vi "fgv_FOV.vi"(8 "error in":errorcluster, 11 "Function":T2) -> (0 "error out":errorcluster, 1 "Objectives (section names)":string[](array[string]), 2 "Data (Format B)":cluster{"FOV setup":T1}[](array[cluster]), 3 "Data (Format A)":T3(array[cluster]))   [LabVIEW 2020]
uses:
  Typedefs/FOV FGV states.ctl
  <vilib>/Utility/miscctls.llb/LVStringsAndValuesArrayTypeDef_SGL.ctl
  Typedefs/Which path.ctl
  <vilib>/Utility/config.llb/Read Key (Double).vi
  <vilib>/Utility/config.llb/NI_LVConfig.lvlib
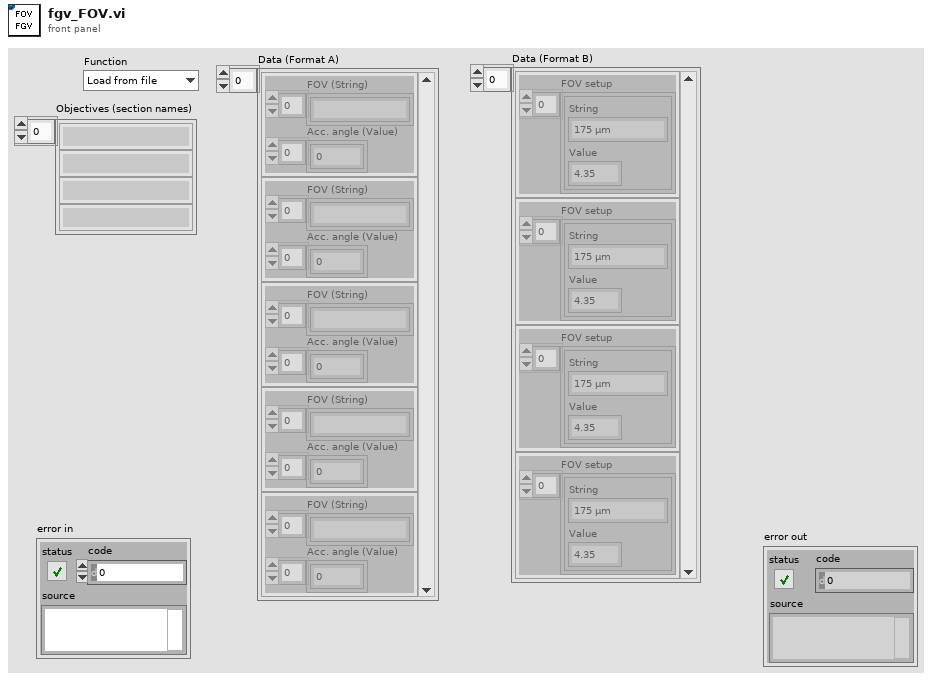
[diagram p1: front panel]
types:
  T1 = typedef "LVStringsAndValuesArrayTypeDef_SGL.ctl" = cluster{"String":string, "Value":sgl}[]
  T2 = typedef "FOV FGV states.ctl" = enum16{"Load from file", "Read FGV", "Update section name", "Delete section", "Add section", "Cleanup ini file"}
  T3 = cluster{"FOV (String)":string[], "Acc. angle (Value)":dbl[]}[]
  T4 = typedef "Which path.ctl" = enum16{"Configuration Files", "Calibration Files", "Images", "Setup.ini", "Loaded User profile.ini", "User's-Previous session.ini", "New user profile.ini", "Selected User profile.ini", "User profiles folder", "Power meter scaling.txt", "FOV Cal.ini", "Calibration.ini"}
  T5 = typedef "NI_LVConfig.lvlib/Config Data RefNum.ctl" = refnum<k1>
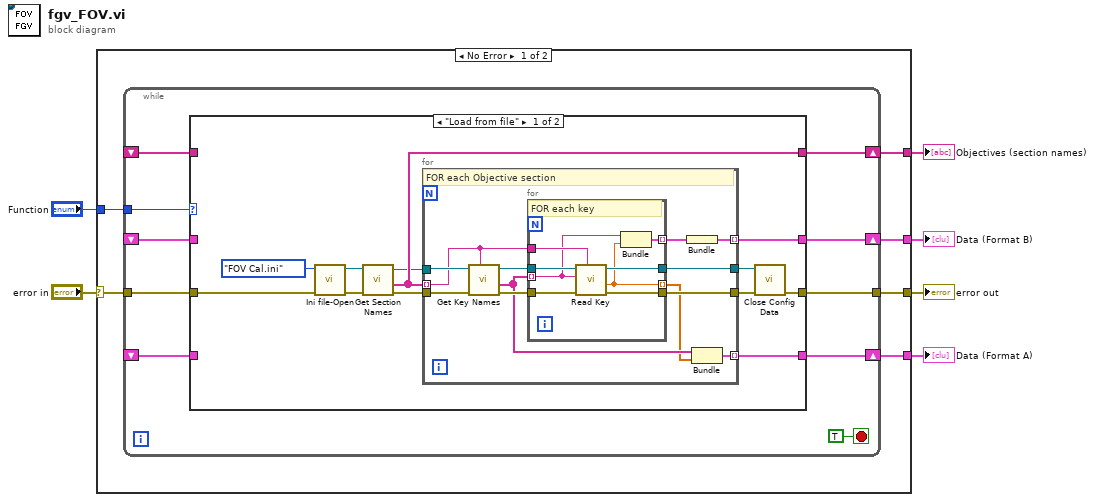
[diagram p0: block diagram]
diagram:
  n1 = case shown="No Error" "error in" {
    selector: "error in" -> [w8 w59]
    tunnel: "Function" -> [w12 _]
    tunnel: [w11 _] -> w5
    tunnel: [w10 _] -> w4
    tunnel: [w9 w59] -> w2
    tunnel: [w7 _] -> w1
    frame No Error {
      n2 = while {
        shift-right: [w22] -> w10
        shift-left: _ -> [w18]
        shift-right: [w21] -> w11
        shift-left: _ -> [w17]
        tunnel: w12 -> [w19]
        tunnel: [w16] -> w9
        tunnel: w8 -> [w15]
        shift-right: [w14] -> w7
        shift-left: _ -> [w13]
        stop <- TRUE stop-if-true
        n3 = case shown="\"Load from file\"" w19 {
          tunnel: [w34 w58] -> w22
          tunnel: [w31 w57] -> w21
          tunnel: w18 -> [_ w58]
          tunnel: w17 -> [_ w57]
          tunnel: [w25 w56] -> w16
          tunnel: w15 -> [w24 w56]
          tunnel: [w23 w55] -> w14
          tunnel: w13 -> [_ w55]
          frame "Load from file" {
            n4 = call "Ini file-Open.vi"("Error In"=w24, "Which file?"=Which_path."FOV Cal.ini") -> ("error out"=w29:errorcluster, "User profile ini file ref"=w28:T5)  [unwired: 6 in, 2 out]
            n5 = call <vilib>:"Get Section Names.vi"("error in (no error)"=w29, "refnum"=w28) -> ("error out"=w32:errorcluster, "section names"=w34:string[], "refnum out"=w33:T5)  [unwired: 7 in]
            n6 = for {
              tunnel: w34 -> [w42] mode=indexing
              tunnel: w33 -> [w46]
              tunnel: [w43] -> w27
              tunnel: w32 -> [w44]
              tunnel: [w40] -> w26
              tunnel: [w37] -> w31 mode=indexing
              tunnel: [w35] -> w23 mode=indexing
              # "FOR each Objective section"
              n7 = call <vilib>:"Get Key Names.vi"("section"=w42, "error in (no error)"=w44, "refnum"=w46) -> ("error out"=w41:errorcluster, "key names"=w39:string[], "refnum out"=w45:T5)  [unwired: 5 in, 1 out]
              n8 = for {
                tunnel: w45 -> [w54]
                tunnel: [w53] -> w43
                tunnel: w42 -> [w52]
                tunnel: w41 -> [w51]
                tunnel: [w50] -> w40
                tunnel: w39 -> [w49] mode=indexing
                tunnel: [w48] -> w38 mode=indexing
                tunnel: [w47] -> w36 mode=indexing
                # "FOR each key"
                n9 = call-poly <vilib>:"Read Key.vi"("section"=w52, "error in (no error)"=w51, "key"=w49, "refnum"=w54) -> ("error out"=w50:errorcluster, "value"=w48:dbl, "refnum out"=w53:T5)  [unwired: 4 in, 1 out]
                n10 = Bundle("String"=w49, "value"=w48) -> (w47:cluster{"String":string, "value":dbl})  [unwired: 1 in]
              }
              n11 = Bundle(w36) -> (w35:cluster{cluster{"String":string, "value":dbl}[]})  [unwired: 1 in]
              n12 = Bundle("key names"=w39, w38) -> (w37:cluster{"key names":string[], dbl[]})  [unwired: 1 in]
            }
            n13 = call <vilib>:"Close Config Data.vi"("error in (no error)"=w26, "refnum"=w27) -> ("error out"=w25:errorcluster)  [unwired: 8 in, 1 out]
          }
          frame "Read FGV", Default {
          }
        }
      }
    }
    frame Error {
    }
  }
  "Objectives (section names)" <- w4
  "Data (Format A)" <- w5
  "error out" <- w2
  "Data (Format B)" <- w1
